vi "zmq_recv.vi"(5 "no block? (F)":bool, 6 "error in":errorcluster, 9 "socket in":refnum<class "zmq_socket.lvclass">) -> (0 "error out":errorcluster, 1 "more?":bool, 2 "data":string, 3 "socket out":refnum<class "zmq_socket.lvclass">, 4 "timeout?":bool)   [LabVIEW 2020, in "zeromq.lvlib" / "zmq_socket.lvclass"]
doc: "Receive a message from the socket and returns the received data as a LabVIEW string (which may contain NULL). If receiving a multi-part message, this VI must be called for each part of the message, and it is the user's obligation to check if this is required. Alternatively, use the zmq_recv_multi VI, which handles this automatically.\n\nIf <b>no block?</b> is True, the function call will return immediately. Use zmq_check_timeout to see if it was simply a timeout or an error occurred.\n\nOtherwise this call will block until a message is received, an error is raised, or the socket is closed.\n\nDetailed API documentation: http://api.zeromq.org/3-2:zmq-recv"
uses:
  zmq_socket.lvclass
  zmq_socket.lvclass/zmq_socket.ctl
  Error Cluster From Error Code.vi
  zeromq.lvlib
panel:
  # "ØMQ"
  # "labview"
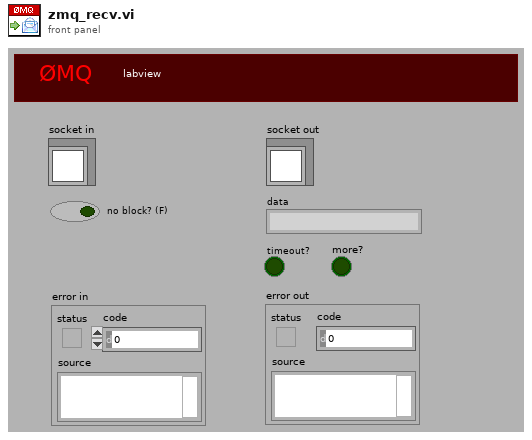
[diagram p1: front panel]
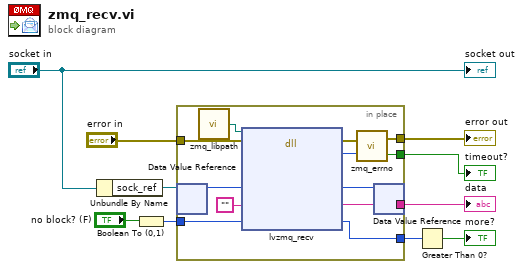
[diagram p0: block diagram]
diagram:
  n1 = Unbundle By Name("socket in") -> ("sock_ref"=w2:refnum<data-value>)
  n2 = Boolean To (0,1)(Boolean="no block? (F)") -> (0, 1=w9:i16)
  n3 = in-place {
    in-place-border: [w20] -> w10
    in-place-border: w9 -> [w19]
    in-place-border: [w18] -> w1
    in-place-border: "error in" -> [w17]
    in-place-border: [w16] -> w6
    in-place-border: [w15] -> w5
    n4 = in-place-dvr #1(w2) -> (w14:u64)  [unwired: 1 out]
    n5 = call "zmq_libpath.vi"() -> ("path"=w11:path)
    n6 = dll-call lib="C:/dev/projs/labview/zeromq3/lvzmq32.dll" fn="lvzmq_recv" ("zmq_labview.dll:lvzmq_socket")(path in=w11, error in=w17, "sock_obj"=w14, "data"="", "flags"=w19) -> (error out=w22:errorcluster, "return type"=w21:i32, "sock_obj"=w13:u64, "data"=w18:string, "flags"=w15:i32)  [unwired: 3 in, 1 out]
    n7 = call "zmq_errno.vi"("retval"=w21, "error in"=w22) -> ("again?"=w20:bool, "error out"=w16:errorcluster)
    n8 = in-place-dvr #1(w13) -> ()  [unwired: 2 out]
  }
  "data" <- w1
  "error out" <- w6
  "timeout?" <- w10
  n9 = Greater Than 0?(x=w5) -> (x > 0?=→"more?":bool)
  "socket out" <- "socket in"
